vi "Utility Short Switch.vi"(0 "VISA resource name":refnum<visa-resource-name>, 5 "Short (F:Off)":bool, 7 "Short Mode (T: Toggle)":bool=TRUE, 11 "error in (no error)":errorcluster) -> (4 "VISA resource name out":refnum<visa-resource-name>, 15 "error out":errorcluster)   [LabVIEW 2015, in "Chroma ATE 6310.lvlib"]
doc: "This function enables/disables the short-circuited simulation,and sets the mode of short key in the electronic load."
uses:
  <instrlib>/Chroma ATE 6310/Chroma ATE 6310.lvlib
panel:
  # "Toggle\nHold"
  # "On\nOff"
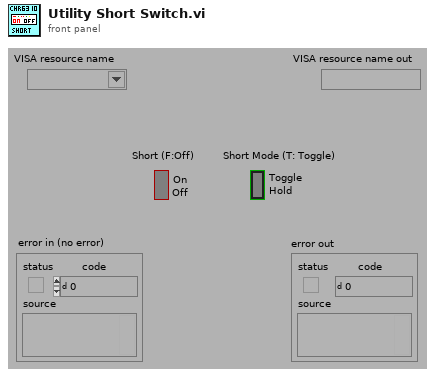
[diagram p1: front panel]
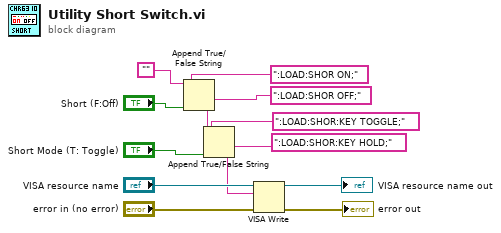
[diagram p0: block diagram]
diagram:
  n1 = Append True/False String(1:"Short (F:Off)", 2:":LOAD:SHOR OFF;", 3:":LOAD:SHOR ON;", 4:"") -> (0:w3:string)
  n2 = Append True/False String(1:"Short Mode (T: Toggle)", 2:":LOAD:SHOR:KEY HOLD;", 3:":LOAD:SHOR:KEY TOGGLE;", 4:w3) -> (0:w1:string)
  n3 = VISA Write(VISA resource name="VISA resource name", write buffer=w1, error in (no error)="error in (no error)") -> (VISA resource name out=→"VISA resource name out":refnum<visa-resource-name>, error out=→"error out":errorcluster)  [unwired: 1 out]
